vi "Read Configuration.vi"(8 "error in (no error)":errorcluster, 11 "Test Runner Spawner In":refnum<class "Test Runner.lvclass">) -> (0 "error out":errorcluster, 3 "Test Runner Spawner Out":refnum<class "Test Runner.lvclass">)   [LabVIEW 2020, in "Test Runner.lvclass"]
doc: "Method that read any necessay configurations from config file or potentially configure hard coded values. The specified configuration file is validated and loaded."
uses:
  Test Runner.lvclass
  C:/Users/anton/Documents/GitHub/LUnit/source/Application Framework/Process Classes/Process/Process.lvclass
  Test Runner.lvclass/Test Runner.ctl
  Application Framework/Process Classes/Process/Process.lvclass
  Application Framework/Support/Configuration File/Configuration File.lvlib
  C:/Users/anton/Documents/GitHub/LUnit/source/Framework/Test Runner/Test Runner.lvclass
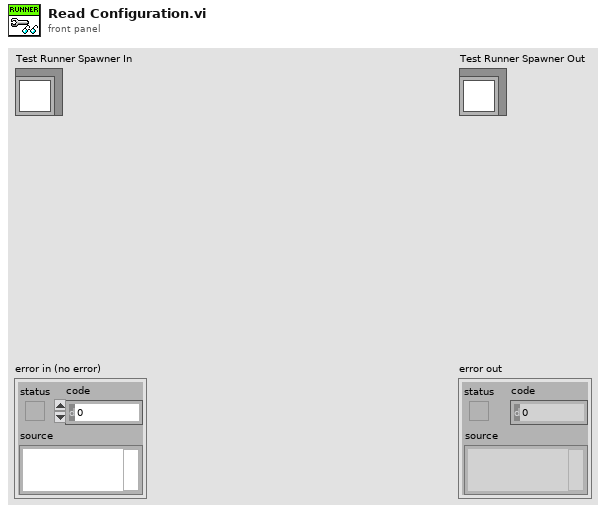
[diagram p1: front panel]
types:
  T1 = typedef "NI_LVConfig.lvlib/Config Data RefNum.ctl" = refnum<k1>
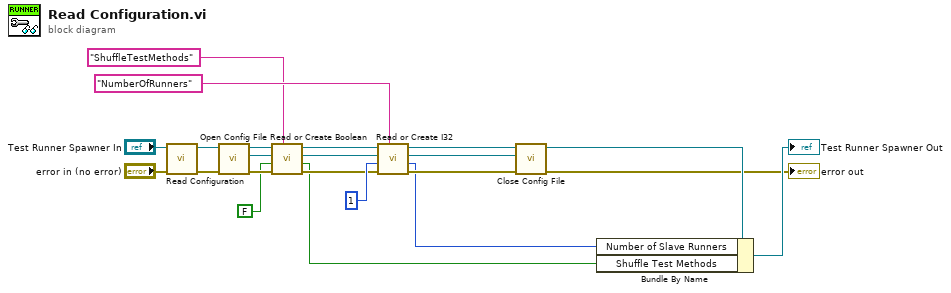
[diagram p0: block diagram]
diagram:
  n1 = call-parent "Read Configuration.vi"("error in (no error)"="error in (no error)", "Process In"="Test Runner Spawner In") -> ("error out"=w12:errorcluster, "Process Out"=w22:refnum<class "Test Runner.lvclass">)  [unwired: 8 in]
  n2 = call "Open Config File.vi"("error in (no error)"=w12, "Process in"=w22) -> ("error out"=w10:errorcluster, "refnum out"=w11:T1, "Process out"=w14:refnum<class "Test Runner.lvclass">)  [unwired: 6 in, 1 out]
  n3 = call "Read or Create Boolean.vi"("key"="ShuffleTestMethods", "error in (no error)"=w10, "default value"=FALSE, "refnum"=w11, "Process in"=w14) -> ("error out"=w8:errorcluster, "value"=w4:bool, "refnum out"=w9:T1, "Process out"=w15:refnum<class "Test Runner.lvclass">)  [unwired: 3 in]
  n4 = call "Read or Create I32.vi"("key"="NumberOfRunners", "error in (no error)"=w8, "default value"=1, "refnum"=w9, "Process in"=w15) -> ("error out"=w6:errorcluster, "value"=w1:i32, "refnum out"=w7:T1, "Process out"=w19:refnum<class "Test Runner.lvclass">)  [unwired: 3 in]
  n5 = call "Close Config File.vi"("error in (no error)"=w6, "refnum"=w7, "Process in"=w19) -> ("error out"=→"error out":errorcluster, "Process out"=w3:refnum<class "Test Runner.lvclass">)  [unwired: 6 in, 1 out]
  n6 = Bundle By Name(cluster=w3, "Number of Slave Runners"=w1, "Shuffle Test Methods"=w4) -> (→"Test Runner Spawner Out":refnum<class "Test Runner.lvclass">)
